vi "validate line configuration.vi"(7 "Module Config":refnum<class "Multiplexer configuration.lvclass">, 11 "Mappings in":T1) -> (1 "valid?":bool, 2 "errors":string, 3 "Mappings out":T1)   [LabVIEW 2021, in "Multiplexer editor node.lvclass"]
doc: "This VI validates modifications to the table of lines and returns any errors as strings."
uses:
  Multiplexer editor node.lvclass
  Mappings.ctl
  <vilib>/NI/Tag Bus Module Framework/channel/TBM channel.lvclass
  C:/Program Files (x86)/National Instruments/LabVIEW 2021/vi.lib/NI/Tag Bus/tag/tag descriptor.lvclass
  configuration/Line.ctl
  Map.ctl
  configuration/Multiplexer configuration.lvclass
  <vilib>/NI/Tag Bus/tag/tag descriptor.lvclass/tag descriptor.ctl
  <vilib>/NI/Tag Bus/tag/read tag name.vi
  <vilib>/NI/Tag Bus/tag/read data type.vi
  Multiplexer editor node.lvclass/Multiplexer editor node.ctl
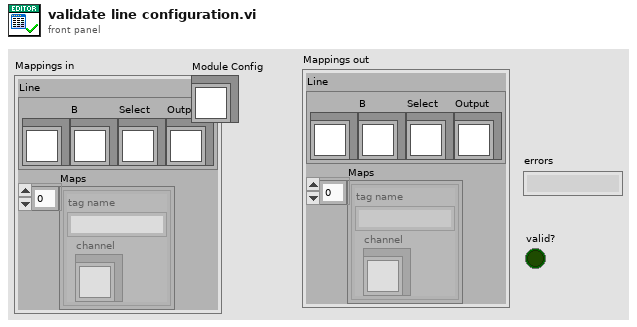
[diagram p1: front panel]
types:
  T1 = typedef "Multiplexer editor node.lvclass/Mappings.ctl" = cluster{"Line":T2, "Maps":T3[]}
  T2 = typedef "Multiplexer configuration.lvclass/Line.ctl" = cluster{"A":refnum<class "TBM channel.lvclass">, "B":refnum<class "TBM channel.lvclass">, "Select":refnum<class "TBM channel.lvclass">, "Output":refnum<class "TBM channel.lvclass">}
  T3 = typedef "Multiplexer editor node.lvclass/Map.ctl" = cluster{"channel":refnum<class "TBM channel.lvclass">, "tag name":string}
  T4 = typedef "tag bus.lvlib/tag descriptor.lvclass/Data Type.ctl" = enum16{"Double", "Single", "I64", "I32", "I16", "I8", "U64", "U32", "U16", "U8", "Boolean", "String", "Array of Double", "Array of Single", "Array of I64", "Array of I32", "Array of I16", "Array of I8", "Array of U64", "Array of U32", "Array of U16", "Array of U8", "Array of Boolean", "Array of String"}
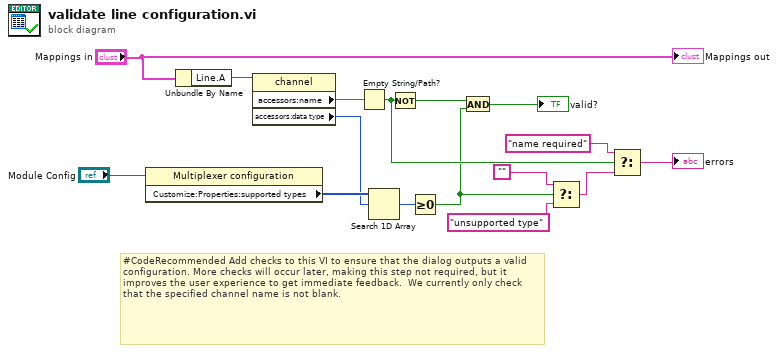
[diagram p0: block diagram]
diagram:
  # "#CodeRecommended Add checks to this VI to ensure that the dialog outputs a valid configuration. More checks will occur later, making this step not required, but it improves the user experience to get immediate feedback.  We currently only check that the specified channel name is not blank."
  n1 = property class="Multiplexer configuration"(reference="Module Config") -> ("Customize:Properties:supported types"=w11:T4[])  [unwired: 1 in, 2 out]
  n2 = Unbundle By Name("Mappings in") -> ("Line.A"=w15:refnum<class "TBM channel.lvclass">)
  n3 = property class="channel"(reference=w15) -> ("accessors:name"=w14:string, "accessors:data type"=w10:T4)  [unwired: 1 in, 2 out]
  n4 = Empty String/Path?(string/path=w14) -> (empty?=w7:bool)
  n5 = Search 1D Array(1D array=w11, element=w10) -> (index of element=w8:i32)  [unwired: 1 in]
  n6 = Not(x=w7) -> (.not. x?=w13:bool)
  n7 = Greater Or Equal To 0?(x=w8) -> (x >= 0?=w4:bool)
  n8 = And(x=w13, y=w4) -> (x .and. y?=→"valid?":bool)
  n9 = Select(t="", s=w4, f="unsupported type") -> (s? t:f=w2:string)
  n10 = Select(t="name required", s=w7, f=w2) -> (s? t:f=→"errors":string)
  "Mappings out" <- "Mappings in"
